vi "Enable or Disable Control.vi"(1 "Enable? (T)":bool) -> (0 "Enable\\Disable":T1(ring))   [LabVIEW 2011]
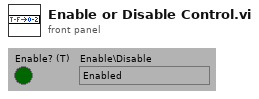
[diagram p1: front panel]
types:
  T1 = enum8{"Enabled", "Disabled", "Disabled and Grayed Out"}
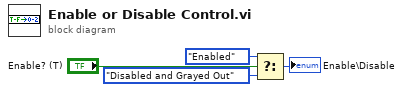
[diagram p0: block diagram]
diagram:
  n1 = Select(t=T1."Enabled" ("Disabled"), s="Enable? (T)", f=T1."Disabled and Grayed Out" ("Disabled")) -> (s? t:f=→"Enable\\Disable":T1)
